vi "Discover USB Signal Generator Model.vi"(10 "Model In":string) -> (2 "selection":bool)   [LabVIEW 2018]
panel:
  out "size(s)":i32
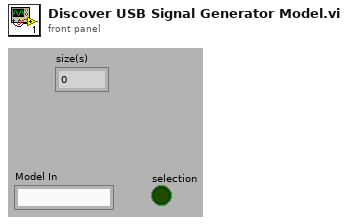
[diagram p1: front panel]
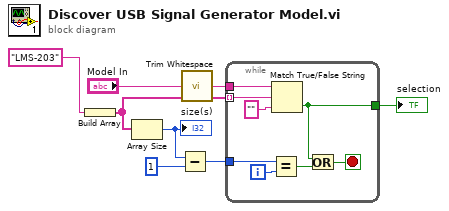
[diagram p0: block diagram]
diagram:
  n1 = Build Array("LMS-203" ("element")) -> (w7:string[])
  n2 = Array Size(array=w7) -> (size(s)=w6:i32)
  "size(s)" <- w6
  n3 = Subtract(x=w6, y=1) -> (x-y=w4:i32)
  n4 = call <vilib>:"Trim Whitespace.vi"("string"="Model In") -> ("trimmed string"=w2:string)  [unwired: 1 in]
  n5 = while {
    tunnel: w7 -> [w15] mode=indexing
    tunnel: w2 -> [w14]
    tunnel: [w13] -> w8
    tunnel: w4 -> [w9]
    i -> [w10]
    stop <- w12 stop-if-true
    n6 = Equal?(x=w9, y=w10) -> (x = y?=w11:bool)
    n7 = Match True/False String(2:"" ("false string"), 3:w15, 4:w14) -> (0:w13:bool)  [unwired: 1 out]
    n8 = Or(x=w13, y=w11) -> (x .or. y?=w12:bool)
  }
  "selection" <- w8
